vi "Write Headers.vi"(8 "error in (no error)":errorcluster, 10 "data":waveform(dbl)[](array[waveform]), 11 "Byte Stream File in":refnum<file>) -> (0 "error out":errorcluster, 3 "Byte Stream File out":refnum<file>)   [LabVIEW 2018, in "CSV Log.lvlib"]
uses:
  CSV Log.lvlib
panel:
  out "Channel Names":string
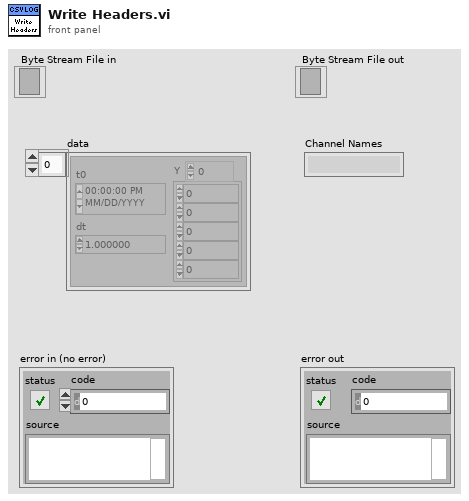
[diagram p1: front panel]
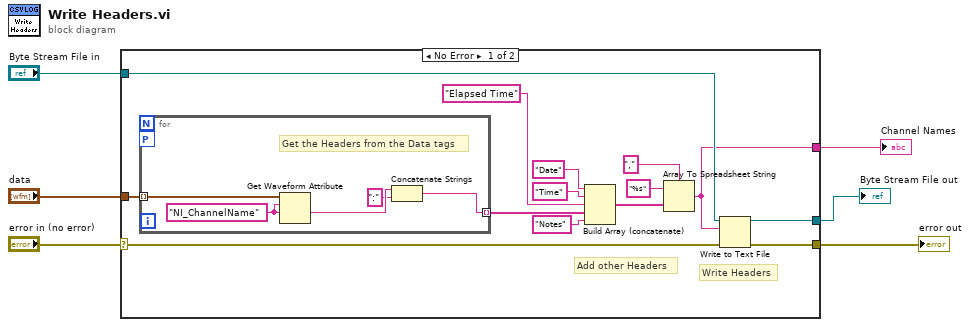
[diagram p0: block diagram]
diagram:
  n1 = case shown="No Error" "error in (no error)" {
    selector: "error in (no error)" -> [w15 w26]
    tunnel: [w14 w26] -> w4
    tunnel: [w17 w27] -> w5
    tunnel: "Byte Stream File in" -> [w16 w27]
    tunnel: "data" -> [w20 _]
    tunnel: [w11 _] -> w1
    frame No Error {
      # "Write Headers"
      # "Add other Headers"
      n2 = for {
        tunnel: w20 -> [w25] mode=indexing
        tunnel: [w21] -> w9 mode=indexing
        workers-P: _ -> [_]
        w24 = "NI_ChannelName" ("name")
        # "Get the Headers from the Data tags"
        n3 = Get Waveform Attribute(5:w24, 6:w24, 7:w25) -> (1:w23:string)  [unwired: 1 in, 3 out]
        n4 = Concatenate Strings(w23, ":" ("string")) -> (w21:string)
      }
      n5 = Build Array (concatenate)("Date", "Time", "Elapsed Time", w9, "Notes" ("element")) -> (w12:string[])
      n6 = Array To Spreadsheet String(delimiter (Tab)=",", array=w12, 3:"%s" ("format string")) -> (spreadsheet string=w11:string)
      n7 = Write to Text File(file (use dialog)=w16, text=w11, error in=w15) -> (refnum out=w17:refnum<file>, error out=w14:errorcluster)  [unwired: 1 in, 1 out]
    }
    frame Error {
    }
  }
  "Byte Stream File out" <- w5
  "error out" <- w4
  "Channel Names" <- w1
